vi "Write Power DVR FIFO Direct Dispatch.vi"(6 "FIFO Timestamps":T1, 8 "error in (no error)":errorcluster, 9 "Timeout (ms)":i32=100, 10 "Data In":refnum<data-value>[](array[refnum]), 11 "CIFTag in":refnum<class "CIFChannels.lvclass">) -> (0 "error out":errorcluster, 1 "timed out?":bool, 2 "Data Out":refnum<data-value>[](array[refnum]), 3 "CIFTag out":refnum<class "CIF_NIChn_Fifo_Power_DVR.lvclass">)   [LabVIEW 2021, in "CIF_NIChn_Fifo_Power_DVR.lvclass"]
uses:
  CIF_NIChn_Fifo_Power_DVR.lvclass
  D:/dev/CIF-LVCore/src/Channels/CIF_NIChn/NIChn/CIF_NIChn.lvclass
  CIFChannels/CIFChannels.lvclass
  ChannelCommon/typedef/TimeStamps.ctl
  ChannelCommon/typedef/Datatype Waveform.ctl
  CIF_NIChn_Fifo_Power_DVR.lvclass/CIF_NIChn_Fifo_Power_DVR.ctl
  ChannelCommon/CIFFIFO/CIFfifo.lvclass/CIFfifo.ctl
  NIChn/CIF_NIChn.lvclass/CIF_NIChn.ctl
  ChannelCommon/CIFFIFO/Accessors/Read Length.vi
  CIFCore/Common/Utilities/Append Error Location.vi
  <vilib>/CIFChannels/SubVIs/Get dll Path.vi
  ChannelCommon/CIFFIFO/Utilities/Update Header.vi
  ChannelCommon/CIFFIFO/Flatten/DVR Flatten.vi
  ChannelCommon/CIFFIFO/Accessors/Write T0.vi
  ChannelCommon/CIFFIFO/Accessors/Write T_Out.vi
  ChannelCommon/CIFFIFO/Accessors/Write ClockID.vi
  ChannelCommon/Utilities/Flatten Header.vi
  ChannelCommon/CIFFIFO/Flatten/DVR Flatten.vi/6fdbece9-bad6-4a8e-9bf7-fe1528478dd6.vi
  ChannelCommon/CIFFIFO/Accessors/Write Payload Length.vi
  ChannelCommon/CIFFIFO/Accessors/Read Header.vi
  CIFCore/Common/Utilities/Add Error.vi
  ChannelCommon/CIFFIFO/Flatten/DVR Flatten.vi/6fdbece9-bad6-4a8e-9bf7-fe1528478dd6.vi/c28b0ead-42ad-4072-80a2-aca7f2bd7ce3.vi
  ChannelCommon/Utilities/Update Time.vi
  NIChn/CIF_NIChn.lvclass
  <vilib>/CIFChannels/CIFChannelCore.lvlib
  ChannelCommon/CIFFIFO/CIFfifo.lvclass
  D:/dev/CIF-LVCore/src/Channels/CIFChannels/CIFChannels.lvclass
  D:/dev/CIF-LVCore/src/Channels/CIF_NIChn/FIFO_Power_DVR/CIF_NIChn_Fifo_Power_DVR.lvclass
  ChannelCommon/ChannelCommon.lvlib
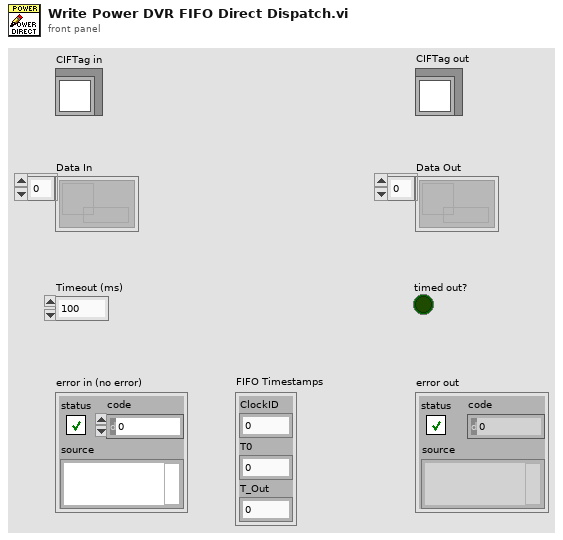
[diagram p1: front panel]
types:
  T1 = typedef "ChannelCommon.lvlib/TimeStamps.ctl" = cluster{"ClockID":u8, "T0":u64, "T_Out":u64}
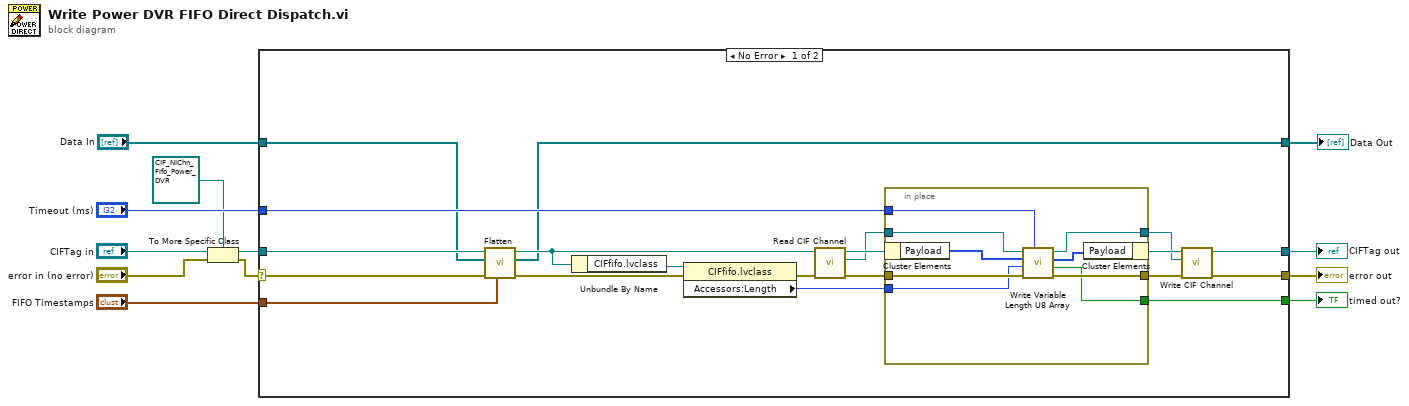
[diagram p0: block diagram]
diagram:
  n1 = To More Specific Class(target class=refnum<class "CIF_NIChn_Fifo_Power_DVR.lvclass"> refnum ("CIFTag in"), reference="CIFTag in", error in="error in (no error)") -> (specific class reference=w6:refnum<class "CIF_NIChn_Fifo_Power_DVR.lvclass">, error out=w3:errorcluster)
  n2 = case shown="No Error" w3 {
    selector: w3 -> [w27 w44]
    tunnel: [w29 w44] -> w12
    tunnel: [w31 w43] -> w11
    tunnel: w6 -> [w28 w43]
    tunnel: [w32 _] -> w10
    tunnel: "Timeout (ms)" -> [w30 _]
    tunnel: "Data In" -> [w14 w42]
    tunnel: [w13 w42] -> w1
    tunnel: "FIFO Timestamps" -> [w26 _]
    frame No Error {
      n3 = call "Flatten.vi"("FIFO Timestamps"=w26, "error in (no error)"=w27, "Data In"=w14, "CIFTag in"=w28) -> ("error out"=w16:errorcluster, "Data Out"=w13:refnum<data-value>[], "CIFTag out"=w17:refnum<class "CIF_NIChn_Fifo_Power_DVR.lvclass">)  [unwired: 5 in]
      n4 = Unbundle By Name(w17) -> ("CIFfifo.lvclass"=w19:refnum<class "CIFfifo.lvclass">)
      n5 = property class="CIFfifo.lvclass"(reference=w19, error in=w16) -> (error out=w18:errorcluster, "Accessors:Length"=w15:u64)  [unwired: 1 out]
      n6 = call "Read CIF Channel.vi"("error in (no error)"=w18, "CIFTag in"=w17) -> ("error out"=w24:errorcluster, "CIF Channel"=w21:refnum<k21>, "CIFTag out"=w25:refnum<class "CIF_NIChn_Fifo_Power_DVR.lvclass">)  [unwired: 7 in]
      n7 = in-place {
        in-place-border: w24 -> [w41]
        in-place-border: [w40] -> w22
        in-place-border: [w39] -> w32
        in-place-border: w21 -> [w38]
        in-place-border: [w37] -> w20
        in-place-border: w30 -> [w36]
        in-place-border: w15 -> [w34]
        n8 = in-place-cluster #1(w25) -> ("Payload"=w35:u8[])
        n9 = call <vilib>:"Write Variable Length U8 Array.vi"("Timeout (ms)"=w36, "error in"=w41, "numElements"=w34, "U8 Array in"=w35, "CIF Channel in"=w38) -> ("error out"=w40:errorcluster, "Timed out?"=w39:bool, "U8 Array out"=w33:u8[], "CIF Channel out"=w37:refnum<k21>)  [unwired: 3 in]
        n10 = in-place-cluster #1("Payload"=w33) -> (w23:refnum<class "CIF_NIChn_Fifo_Power_DVR.lvclass">)
      }
      n11 = call "Write CIF Channel.vi"("error in (no error)"=w22, "CIF Channel"=w20, "CIFTag in"=w23) -> ("error out"=w29:errorcluster, "CIFTag out"=w31:refnum<class "CIF_NIChn_Fifo_Power_DVR.lvclass">)  [unwired: 7 in]
    }
    frame Error {
    }
  }
  "error out" <- w12
  "CIFTag out" <- w11
  "timed out?" <- w10
  "Data Out" <- w1
